vi "Infer Control Type.vi"(8 "error in (no error)":errorcluster, 10 "Ctl Refnum":refnum<vi>, 11 "Editor in":refnum<class "Editor.lvclass">) -> (0 "error out":errorcluster, 2 "Control Type":string, 3 "Editor out":refnum<class "Editor.lvclass">)   [LabVIEW 2020, in "VolatusGUIEditor.lvlib" / "Editor.lvclass"]
uses:
  Editor.lvclass
  Editor.lvclass/Editor.ctl
  ControlBindingPanel/ControlBindingPanel.lvclass
  C:/dev/lv20CE/relink/lv-oopanel/OOPanel/Panel/Panel.lvclass
  lv-oopanel/OOPanel/Manager/Manager.lvclass
  VolatusGUIControls/VolatusGUIControls.lvlib
  Control List/Control List.lvclass
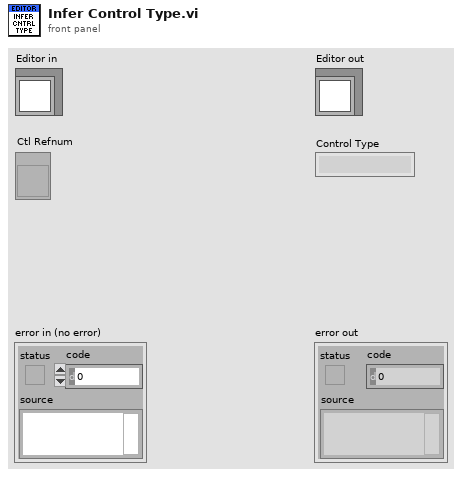
[diagram p1: front panel]
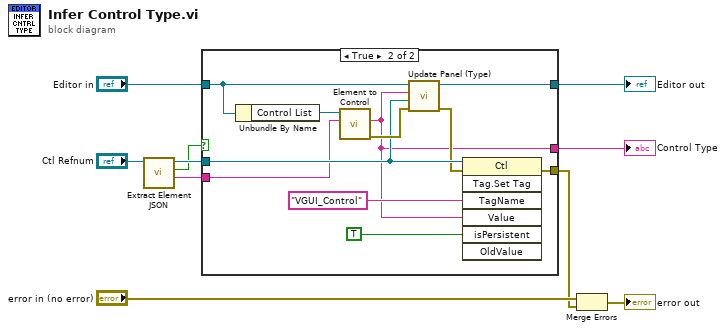
[diagram p0: block diagram]
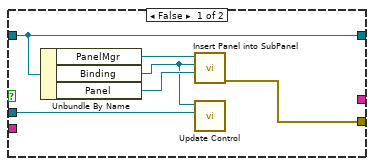
[diagram p2: hidden frame]
diagram:
  n1 = call "Extract Element JSON.vi"("Ctl Refnum in"="Ctl Refnum") -> ("Type"=w6:string, "Is GUI Element"=w4:bool, "Ctl Refnum"=w7:refnum<vi>)  [unwired: 7 in, 1 out]
  n2 = case shown="True" w4 {
    tunnel: "Editor in" -> [w12 w25]
    tunnel: w7 -> [w13 w21]
    tunnel: w6 -> [_ w18]
    tunnel: [w12 w24] -> w5
    tunnel: [w11 w20] -> w2
    tunnel: [_ w17] -> w1
    frame False {
      n3 = Unbundle By Name(w12) -> ("PanelMgr"=w14:refnum<class "Manager.lvclass">, "Binding"=w15:refnum<class "ControlBindingPanel.lvclass">, "Panel"=w16:refnum<vi>)
      n4 = call "Insert Panel into SubPanel.vi"("SubPanel"=w16, "Panel In"=w15, "Manager in"=w14) -> ("error out"=w11:errorcluster)  [unwired: 6 in, 2 out]
      n5 = call "Update Control.vi"("Ctl Refnum"=w13, "ControlBindingPanel in"=w15) -> ()  [unwired: 8 in, 2 out]
    }
    frame True {
      n6 = Unbundle By Name(w25) -> ("Control List"=w26:refnum<class "Control List.lvclass">)
      n7 = call "Element to Control.vi"("Element Type"=w18, "Control List in"=w26) -> ("error out"=w27:errorcluster, "Control Type"=w17:string)  [unwired: 7 in, 1 out]
      n8 = call "Update Panel (Type).vi"("error in (no error)"=w27, "Ctl Refnum"=w21, "Control Type"=w17, "Editor in"=w25) -> ("error out"=w19:errorcluster, "Editor out"=w24:refnum<class "Editor.lvclass">)  [unwired: 6 in]
      n9 = invoke class="Ctl" method="Tag.Set Tag"(reference=w21, error in=w19, "TagName"="VGUI_Control" ("Tag Name"), "Value"=w17, "isPersistent"=TRUE ("Is Persistent?")) -> (error out=w20:errorcluster)  [unwired: 2 in, 6 out]
    }
  }
  "Editor out" <- w5
  "Control Type" <- w1
  n10 = Merge Errors("error in (no error)", w2) -> (→"error out":errorcluster)
